vi "Get Display Text.vi"(8 "error in (no error)":errorcluster, 11 "Reference in":refnum<class "Reference.lvclass">) -> (0 "error out":errorcluster, 1 "Detail Text":string, 2 "Display Name":string, 3 "Reference out":refnum<class "Reference.lvclass">)   [LabVIEW 2018, in "VILab.lvlib" / "Reference.lvclass"]
uses:
  Reference.lvclass
  C:/Users/Flarn/Documents/LabVIEW Projects/Low-Level VI Manipulation/Support Files/VILab/Element.lvclass
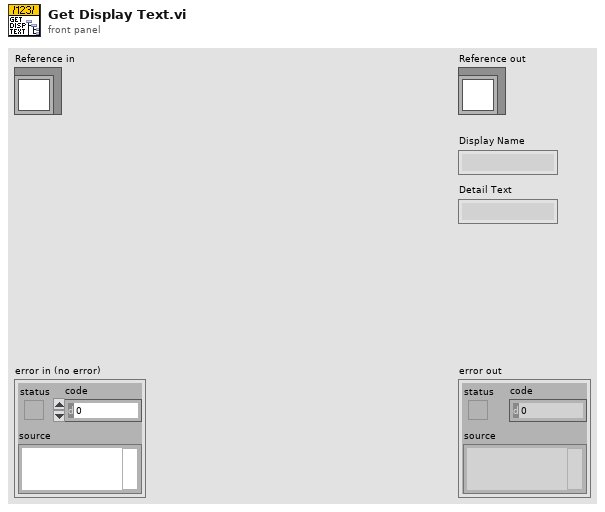
[diagram p1: front panel]
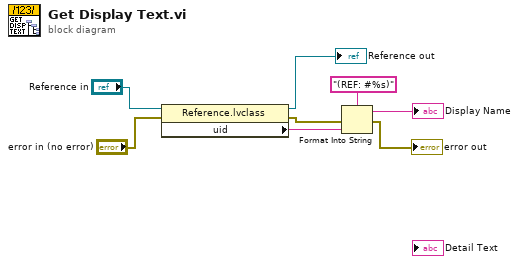
[diagram p0: block diagram]
diagram:
  n1 = property class="Reference.lvclass"(reference="Reference in", error in="error in (no error)") -> (reference out=→"Reference out":refnum<class "Reference.lvclass">, error out=w3:errorcluster, "uid"=w6:string)
  n2 = Format Into String(format string="(REF: #%s)", error in=w3, w6) -> (resulting string=→"Display Name":string, error out=→"error out":errorcluster)  [unwired: 1 in]
